vi "Highlight Assert Node.vi"(8 "error in (no error)":errorcluster, 10 "Assertion Label":string, 11 "vi reference":refnum<vi>) -> (0 "error out":errorcluster, 3 "vi reference  dup":refnum<vi>)   [LabVIEW 2013, in "Caraya.lvlib" / "Basic Test Manager.lvclass"]
uses:
  Basic Test Manager.lvclass
  <vilib>/Utility/traverseref.llb/TRef TravTarget.ctl
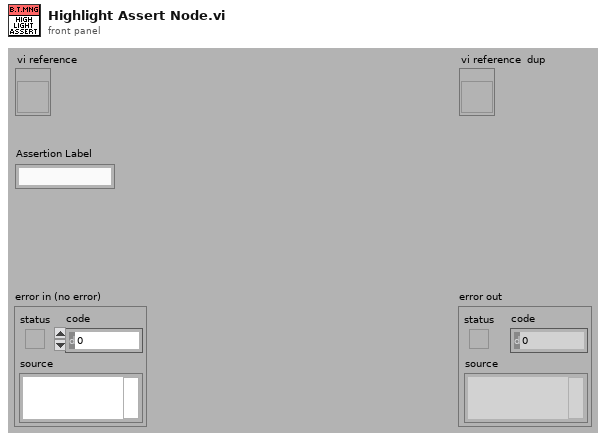
[diagram p1: front panel]
types:
  T1 = typedef "TRef TravTarget.ctl" = enum16{"FP", "BD", "Other"}
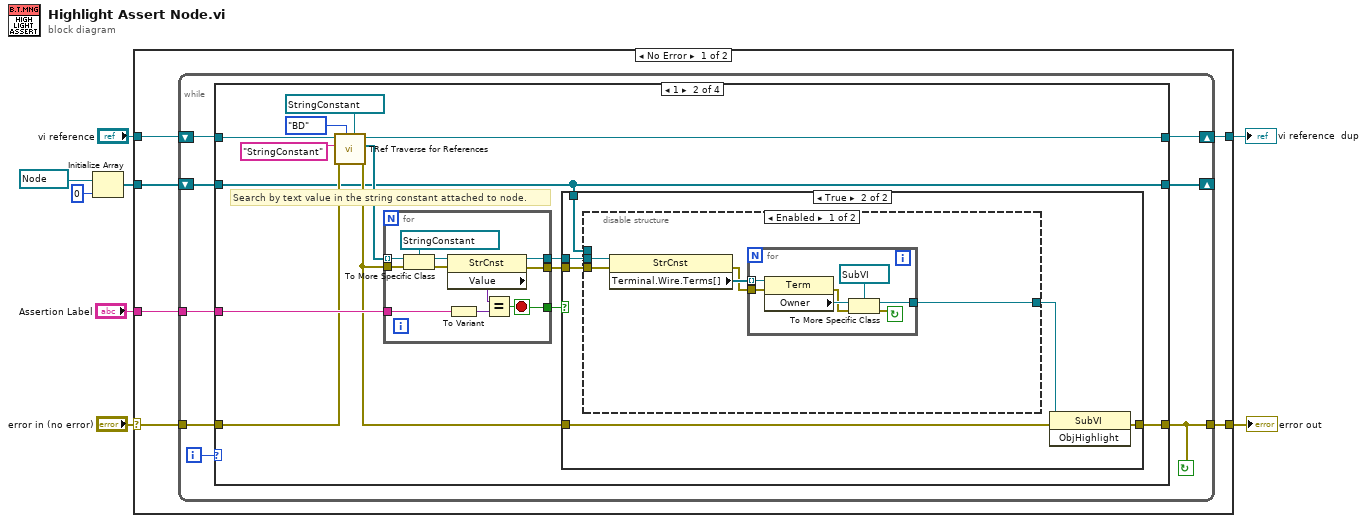
[diagram p0: block diagram]
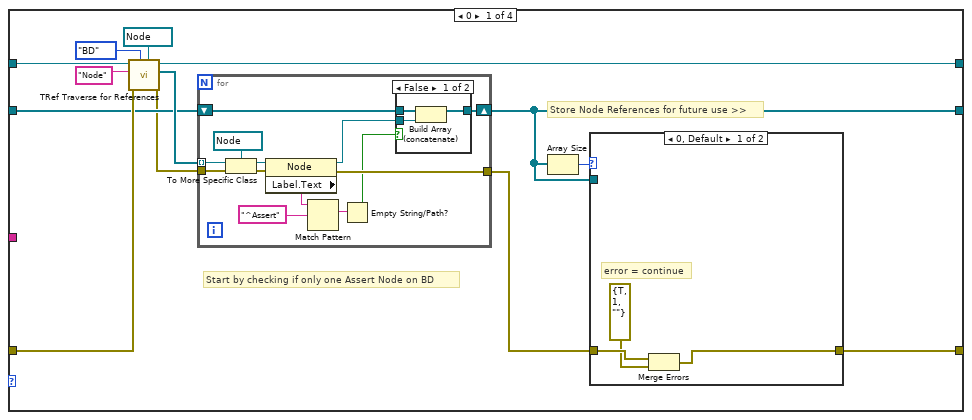
[diagram p2: hidden frame]
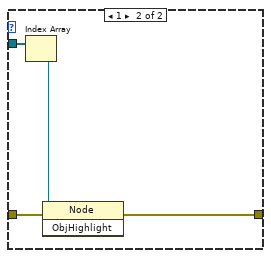
[diagram p3: hidden frame]
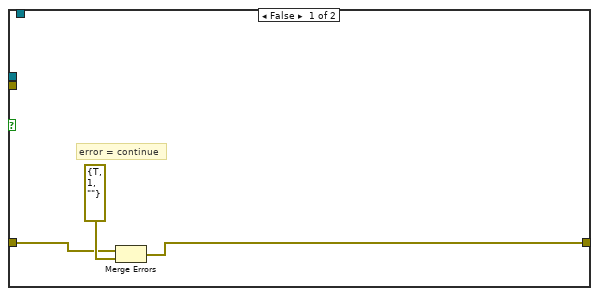
[diagram p5: hidden frame]
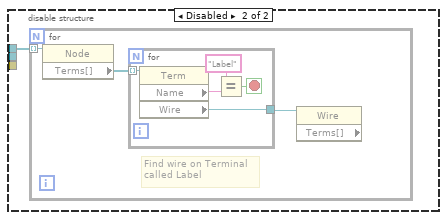
[diagram p6: hidden frame]
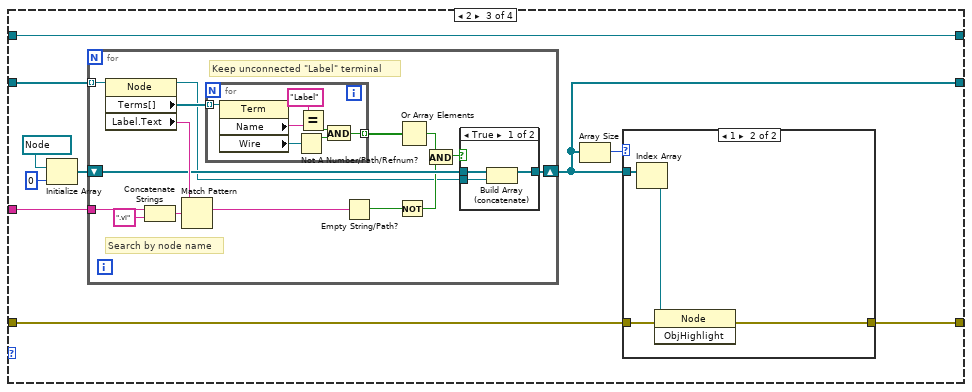
[diagram p7: hidden frame]
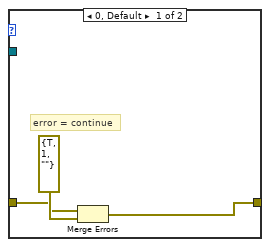
[diagram p8: hidden frame]
diagram:
  n1 = Initialize Array(refnum<vi> refnum ("Other Refnum"), 0 ("dimension size")) -> (w1:refnum<vi>[])
  n2 = case shown="No Error" "error in (no error)" {
    selector: "error in (no error)" -> [w13 w162]
    tunnel: [w11 w162] -> w7
    tunnel: "vi reference" -> [w10 w161]
    tunnel: [w12 w161] -> w5
    tunnel: "Assertion Label" -> [w14 _]
    tunnel: w1 -> [w9 _]
    frame No Error {
      n3 = while {
        tunnel: w14 -> [w22]
        tunnel: w13 -> [w21]
        tunnel: [w15] -> w11
        shift-right: [w20] -> w12
        shift-left: w10 -> [w19]
        shift-right: [w16] -> _
        shift-left: w9 -> [w17]
        i -> [w18]
        stop <- w15 continue-if-true
        n4 = case shown="1" w18 {
          tunnel: w22 -> [_ w69 w124 _]
          tunnel: w21 -> [w33 w67 w121 w159]
          tunnel: [w31 w65 w122 w160] -> w20
          tunnel: [w30 w64 w123 w159] -> w15
          tunnel: w19 -> [w29 w62 w122 w160]
          tunnel: w17 -> [w27 w60 w119 w158]
          tunnel: [w25 w60 w118 w158] -> w16
          frame 0 {
            # "Store Node References for future use >>"
            # "Start by checking if only one Assert Node on BD"
            n5 = call <vilib>:"TRef Traverse for References.vi"("Other Refnum"=refnum<vi> refnum, "Traverse Target"=TRef_TravTarget."BD", "error in (no error)"=w33, "Class Name"="Node", "VI Refnum"=w29) -> ("error out"=w24:errorcluster, "References"=w34:refnum<vi>[], "dup VI Refnum"=w31:refnum<vi>)  [unwired: 3 in, 1 out]
            n6 = for {
              tunnel: w34 -> [w55] mode=indexing
              tunnel: [w51] -> w23
              shift-right: [w44] -> w25
              shift-left: w27 -> [w46]
              tunnel: w24 -> [w43]
              n7 = To More Specific Class(target class=refnum<vi> refnum ("Other Refnum"), reference=w55, error in=w43) -> (specific class reference=w53:refnum<vi>, error out=w52:errorcluster)
              n8 = property class="Node"(reference=w53, error in=w52) -> (reference out=w45:refnum<vi>, error out=w51:errorcluster, "Label.Text"=w50:string)
              n9 = Match Pattern(string=w50, regular expression="^Assert" ("Class Name")) -> (match substring=w48:string)  [unwired: 1 in, 3 out]
              n10 = Empty String/Path?(string/path=w48) -> (empty?=w47:bool)
              n11 = case shown="False" w47 {
                tunnel: w46 -> [w58 w59]
                tunnel: w45 -> [w57 _]
                tunnel: [w56 w59] -> w44
                frame False {
                  n12 = Build Array (concatenate)(w58, w57) -> (w56:refnum<vi>[])
                }
                frame True {
                }
              }
            }
            n13 = Array Size(array=w25) -> (size(s)=w26:i32)
            n14 = case shown="0, Default" w26 {
              tunnel: w23 -> [w38 w42]
              tunnel: [w36 w41] -> w30
              tunnel: w25 -> [_ w40]
              frame 0, Default {
                # "error = continue"
                n15 = Merge Errors(w38, errorcluster {"status"=TRUE, "code"=1, "source"=""} ("error out")) -> (w36:errorcluster)
              }
              frame 1 {
                n16 = Index Array(array=w40) -> (element=w39:refnum<vi>)  [unwired: 1 in]
                n17 = invoke class="Node" method="ObjHighlight"(reference=w39, error in=w42) -> (error out=w41:errorcluster)  [unwired: 1 in, 2 out]
              }
            }
          }
          frame 1 {
            # "Search by text value in the string constant attached to node."
            n18 = call <vilib>:"TRef Traverse for References.vi"("Other Refnum"=refnum<vi> refnum, "Traverse Target"=TRef_TravTarget."BD", "error in (no error)"=w67, "Class Name"="StringConstant", "VI Refnum"=w62) -> ("error out"=w61:errorcluster, "References"=w71:refnum<vi>[], "dup VI Refnum"=w65:refnum<vi>)  [unwired: 3 in, 1 out]
            n19 = for {
              tunnel: w71 -> [w114] mode=indexing
              tunnel: [w110] -> w73
              tunnel: w69 -> [w108]
              tunnel: [w107] -> w68
              tunnel: [w105] -> w63
              tunnel: w61 -> [w104]
              stop <- w105 stop-if-true
              n20 = To More Specific Class(target class=refnum<vi> refnum ("Other Refnum"), reference=w114, error in=w104) -> (specific class reference=w112:refnum<vi>, error out=w111:errorcluster)
              n21 = property class="StrCnst"(reference=w112, error in=w111) -> (reference out=w110:refnum<vi>, error out=w107:errorcluster, "Value"=w109:variant)
              n22 = To Variant(anything=w108) -> (Variant=w106:variant)
              n23 = Equal?(x=w109, y=w106) -> (x = y?=w105:bool)
            }
            n24 = case shown="True" w63 {
              tunnel: w73 -> [_ w82]
              tunnel: w68 -> [_ w80]
              tunnel: w61 -> [w75 w79]
              tunnel: [w74 w78] -> w64
              tunnel: w60 -> [_ w77]
              frame False {
                # "error = continue"
                n25 = Merge Errors(w75, errorcluster {"status"=TRUE, "code"=1, "source"=""} ("error out")) -> (w74:errorcluster)
              }
              frame True {
                n26 = disable-structure shown="Enabled" {
                  disable-tunnel: w82 -> [w83 _]
                  disable-tunnel: [w86 _] -> w81
                  disable-tunnel: w80 -> [w84 _]
                  disable-tunnel: w77 -> [_ w95]
                  frame Enabled {
                    n27 = property class="StrCnst"(reference=w83, error in=w84) -> (error out=w85:errorcluster, "Terminal.Wire.Terms[]"=w87:refnum<vi>[])  [unwired: 1 out]
                    n28 = for {
                      tunnel: w87 -> [w94] mode=indexing
                      tunnel: [w91] -> w86
                      tunnel: w85 -> [w89]
                      stop <- w90 continue-if-true
                      n29 = property class="Term"(reference=w94, error in=w89) -> (error out=w88:errorcluster, "Owner"=w92:refnum<vi>)  [unwired: 1 out]
                      n30 = To More Specific Class(target class=refnum<vi> refnum ("Other Refnum"), reference=w92, error in=w88) -> (specific class reference=w91:refnum<vi>, error out=w90:errorcluster)
                    }
                  }
                  frame Disabled {
                    n31 = for {
                      tunnel: w95 -> [w98] mode=indexing
                      # "Find wire on Terminal\ncalled Label"
                      n32 = property class="Node"(reference=w98) -> ("Terms[]"=w97:refnum<vi>[])  [unwired: 1 in, 2 out]
                      n33 = for {
                        tunnel: w97 -> [w103] mode=indexing
                        tunnel: [w99] -> w96
                        stop <- w100 stop-if-true
                        n34 = property class="Term"(reference=w103) -> ("Name"=w102:string, "Wire"=w99:refnum<vi>)  [unwired: 1 in, 2 out]
                        n35 = Equal?(x="Label" ("string"), y=w102) -> (x = y?=w100:bool)
                      }
                      n36 = property class="Wire" props=["Terms[]"](reference=w96) -> ()  [unwired: 1 in, 3 out]
                    }
                  }
                }
                n37 = invoke class="SubVI" method="ObjHighlight"(reference=w81, error in=w79) -> (error out=w78:errorcluster)  [unwired: 1 in, 2 out]
              }
            }
          }
          frame 2 {
            n38 = Initialize Array(refnum<vi> refnum ("Other Refnum"), 0 ("dimension size")) -> (w116:refnum<vi>[])
            n39 = for {
              tunnel: w119 -> [w146] mode=indexing
              tunnel: w124 -> [w145]
              shift-right: [w140] -> w118
              shift-left: w116 -> [w141]
              # "Keep unconnected \"Label\" terminal"
              # "Search by node name"
              n40 = property class="Node"(reference=w146) -> (reference out=w133:refnum<vi>, "Terms[]"=w134:refnum<vi>[], "Label.Text"=w144:string)  [unwired: 1 in, 1 out]
              n41 = Concatenate Strings(w145, ".vi" ("string")) -> (w142:string)
              n42 = Match Pattern(string=w144, regular expression=w142) -> (match substring=w136:string)  [unwired: 1 in, 3 out]
              n43 = for {
                tunnel: w134 -> [w153] mode=indexing
                tunnel: [w147] -> w139 mode=indexing
                n44 = property class="Term"(reference=w153) -> ("Name"=w152:string, "Wire"=w150:refnum<vi>)  [unwired: 1 in, 2 out]
                n45 = Not A Number/Path/Refnum?(number/path/refnum=w150) -> (NaN/Path/Refnum?=w148:bool)
                n46 = Equal?(x="Label" ("string"), y=w152) -> (x = y?=w149:bool)
                n47 = And(x=w149, y=w148) -> (x .and. y?=w147:bool)
              }
              n48 = Empty String/Path?(string/path=w136) -> (empty?=w138:bool)
              n49 = Not(x=w138) -> (.not. x?=w137:bool)
              n50 = Or Array Elements(Boolean array=w139) -> (logical OR=w132:bool)
              n51 = And(x=w132, y=w137) -> (x .and. y?=w135:bool)
              n52 = case shown="True" w135 {
                tunnel: w141 -> [w156 w157]
                tunnel: [w154 w157] -> w140
                tunnel: w133 -> [w155 _]
                frame True {
                  n53 = Build Array (concatenate)(w156, w155) -> (w154:refnum<vi>[])
                }
                frame False {
                }
              }
            }
            n54 = Array Size(array=w118) -> (size(s)=w120:i32)
            n55 = case shown="1" w120 {
              tunnel: w121 -> [w126 w131]
              tunnel: [w125 w128] -> w123
              tunnel: w118 -> [_ w130]
              frame 0, Default {
                # "error = continue"
                n56 = Merge Errors(w126, errorcluster {"status"=TRUE, "code"=1, "source"=""} ("error out")) -> (w125:errorcluster)
              }
              frame 1 {
                n57 = Index Array(array=w130) -> (element=w129:refnum<vi>)  [unwired: 1 in]
                n58 = invoke class="Node" method="ObjHighlight"(reference=w129, error in=w131) -> (error out=w128:errorcluster)  [unwired: 1 in, 2 out]
              }
            }
          }
          frame Default {
            # "Give up search for node, no more criteria to discriminate"
          }
        }
      }
    }
    frame Error {
    }
  }
  "error out" <- w7
  "vi reference  dup" <- w5
